vi "Check if Refs are Valid.vi"(8 "error in (no error)":errorcluster, 11 "motor communication ref in":refnum<class "NI_Robotics_Motor Communication Ref.lvclass">) -> (0 "error out":errorcluster, 2 "valid?":bool, 3 "motor communication ref out":refnum<class "NI_Robotics_Motor Communication Ref.lvclass">)   [LabVIEW 2017, in "NI_Robotics_Motor Communication Ref.lvclass"]
uses:
  <vilib>/robotics/Actuation/Motor Communication Ref/NI_Robotics_Motor Communication Ref.lvclass
  <vilib>/robotics/Actuation/Motor Communication Ref/NI_Robotics_Motor Communication Ref.lvclass/NI_Robotics_Motor Communication Ref.ctl
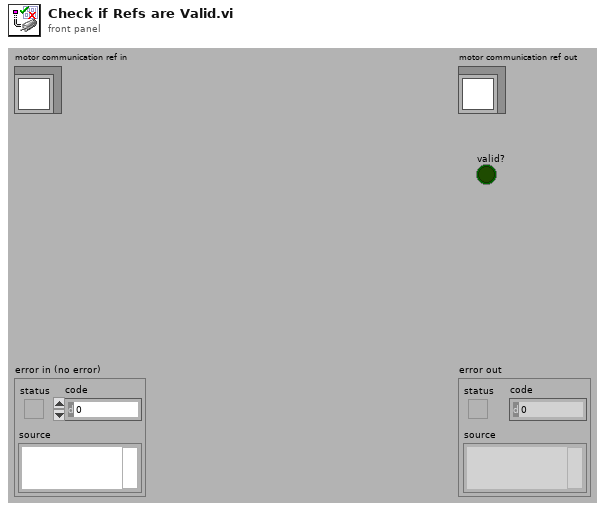
[diagram p1: front panel]
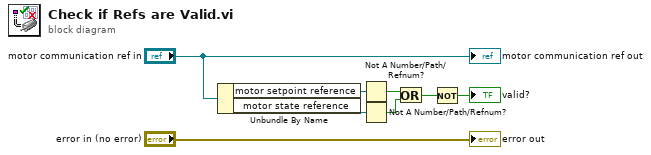
[diagram p0: block diagram]
diagram:
  n1 = Unbundle By Name("motor communication ref in") -> ("motor setpoint reference"=w2:refnum<data-value>, "motor state reference"=w3:refnum<data-value>)
  n2 = Not A Number/Path/Refnum?(number/path/refnum=w2) -> (NaN/Path/Refnum?=w4:bool)
  n3 = Not A Number/Path/Refnum?(number/path/refnum=w3) -> (NaN/Path/Refnum?=w5:bool)
  n4 = Or(x=w4, y=w5) -> (x .or. y?=w6:bool)
  n5 = Not(x=w6) -> (.not. x?=→"valid?":bool)
  "error out" <- "error in (no error)"
  "motor communication ref out" <- "motor communication ref in"
